vi "id.Get ID Type.vi"(8 "error in (no error)":errorcluster, 11 "id in":refnum<class "id.lvclass">) -> (0 "error out":errorcluster, 2 "Type":T1, 3 "id out":refnum<class "id.lvclass">)   [LabVIEW 2017, in "id.lvclass"]
uses:
  id.lvclass
  <vilib>/Utility/Data Type/Type Definitions/Data Type.ctl
  id.lvclass/id.ctl
  <vilib>/Utility/Data Type/NI_Data Type.lvlib
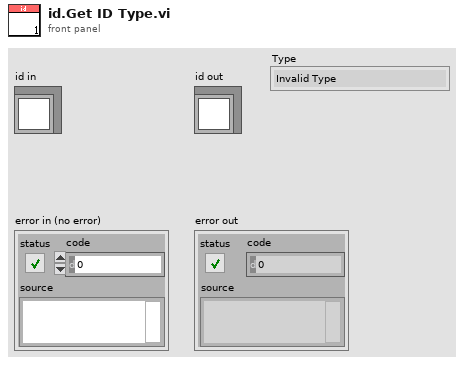
[diagram p1: front panel]
types:
  T1 = typedef "NI_Data Type.lvlib/Data Type.ctl" = enum8{"Invalid Type", "Void", "I8", "I16", "I32", "I64", "U8", "U16", "U32", "U64", "Single Float", "Double Float", "Extended Float", "Single Complex", "Double Complex", "Extended Complex", "Enum U8", "Enum U16", "Enum U32", "Enum U64", "Single Float With Unit", "Double Float With Unit", "Extended Float With Unit", "Single Complex with Unit", "Double Complex with Unit", "Extended Complex with Unit", "Boolean", "String", "Path", "Picture", "Tag", "Array", "Cluster", "Variant", "LV Variant", "Waveform", "Timestamp", "Digital Waveform", "Digital Data", "ExpressData", "Refnum", "External Data", "VI", "Poly VI", "LabVIEW Class Instance", "Fixed Point"}
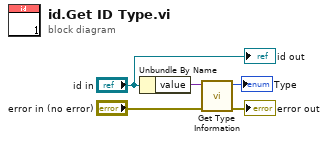
[diagram p0: block diagram]
diagram:
  n1 = Unbundle By Name("id in") -> ("value"=w5:variant)
  n2 = call <vilib>:"Get Type Information.vi"("error in (no error)"="error in (no error)", "Variant"=w5) -> ("error out"=→"error out":errorcluster, "Type"=→"Type":T1)  [unwired: 5 in, 3 out]
  "id out" <- "id in"
